vi "ui_getOffsetMultiplier.vi"(11 "Axis":dbl[](array[numeric])) -> (2 "Multiplier":dbl, 3 "Offset":dbl)   [LabVIEW 2015]
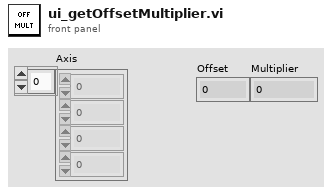
[diagram p1: front panel]
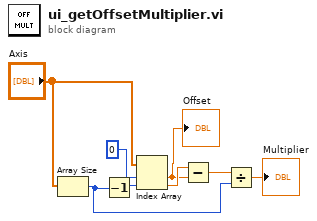
[diagram p0: block diagram]
diagram:
  n1 = Array Size(array="Axis") -> (size(s)=w3:i32)
  n2 = Decrement(x=w3) -> (x-1=w4:i32)
  n3 = Index Array(array="Axis", index #1=0 ("index"), index #2=w4) -> (element #1=w2:dbl, element #2=w7:dbl)
  "Offset" <- w2
  n4 = Subtract(x=w7, y=w2) -> (x-y=w6:dbl)
  n5 = Divide(x=w6, y=w3) -> (x/y=→"Multiplier":dbl)
